vi "PWM Generation.vi"() -> ()   [LabVIEW 2021]
uses:
  <vilib>/myRIO/Instrument Drivers/Onboard IO/DIO/typedefs/DIO Reference.ctl
  <vilib>/myRIO/Common/Instrument Driver Framework/Utilities/typedefs/myRIO Generic Hardware Reference.ctl
  <vilib>/myRIO/Common/Instrument Driver Framework/Utilities/typedefs/Hardware Version Enum.ctl
  <vilib>/myRIO/Common/Instrument Driver Framework/Utilities/typedefs/myRIO v1.0 Reference.ctl
  <vilib>/myRIO/Common/Instrument Driver Framework/Utilities/typedefs/Generic FPGA Reference.ctl
  <vilib>/myRIO/Common/Instrument Driver Framework/myRIO v1.0/DIO/typedefs/DIO Channels List.ctl
  <vilib>/myRIO/Common/Instrument Driver Framework/myRIO v1.0/DIO/typedefs/DIO Channels Enum.ctl
  <vilib>/userDefined/High Color/nirio_resource_hc.ctl
  <vilib>/myRIO/Common/Instrument Driver Framework/Utilities/vis/Is FPGA Ref Available.vi
  <vilib>/myRIO/Common/Instrument Driver Framework/myRIO v1.0/DIO/vis/myRIO v1.1 Open Throughput DIO.vi
  <vilib>/myRIO/Instrument Drivers/Onboard IO/DIO/vis/Write.vi
  <vilib>/myRIO/Common/Instrument Driver Framework/Utilities/vis/Validate Channels.vi
  <vilib>/myRIO/Common/Instrument Driver Framework/myRIO v1.0/DIO/vis/myRIO v1.0 Reserve DIO.vi
  <vilib>/myRIO/Common/Instrument Driver Framework/myRIO v1.0/Resource Manager/vis/myRIO v1.0 Reserve Channel List.vi
  <vilib>/myRIO/Common/Instrument Driver Framework/myRIO v1.0/DIO/vis/myRIO v1.0 Build MUX Configuration DIO.vi
  <vilib>/myRIO/Common/Instrument Driver Framework/myRIO v1.0/Resource Manager/vis/myRIO v1.0 Reserve Channel.vi
  <vilib>/myRIO/Common/Instrument Driver Framework/myRIO v1.0/Resource Manager/vis/myRIO v1.0 Unreserve Channel.vi
  <vilib>/myRIO/Common/Instrument Driver Framework/myRIO v1.0/Resource Manager/vis/myRIO v1.0 Create Configuration List.vi
  <vilib>/myRIO/Common/Instrument Driver Framework/myRIO v1.0/Resource Manager/vis/myRIO v1.0 Build Mutex Name.vi
  <vilib>/Utility/VariantDataType/GetNumericInfo.vi
  <vilib>/Utility/error.llb/Error Cluster From Error Code.vi
  <vilib>/myRIO/Common/Instrument Driver Framework/myRIO v1.0/myRIO v1.1 Open Throughput.vi
  <vilib>/myRIO/Common/Instrument Driver Framework/Utilities/vis/IO Manager.vi
  <vilib>/myRIO/Common/Instrument Driver Framework/Utilities/vis/Configuration Manager.vi
  <vilib>/myRIO/Common/Instrument Driver Framework/myRIO v1.0/Resource Manager/vis/myRIO v1.0 Configure IO.vi
  <vilib>/myRIO/Common/Instrument Driver Framework/myRIO v1.0/myRIO v1.0 Close.vi
  <vilib>/myRIO/Common/Instrument Driver Framework/myRIO v1.0/DIO/vis/myRIO v1.0 Write DIO.vi
  <vilib>/myRIO/Express VI/Onboard Devices/LED/LED Express VI.xnode
  <vilib>/myRIO/Instrument Drivers/Onboard IO/DIO/vis/myRIO DIO Open.xnode
  <vilib>/myRIO/Instrument Drivers/Onboard IO/DIO/DIO.lvlib
panel:
  out "?":bool
  out "?":dbl format="%#_2g"
  out "?":bool
  in  "?":bool
  in  "?":u32=100
  in  "Duty Cycle (%) for PWM 2":dbl(slide)=50.0 caption="Duty Cycle (%)" scale=0.0..100.0
  in  "Frequency for PWM 2":dbl(slide)=10.1 caption="Frequency" scale=0.0..100.0
  in  "Duty Cycle (%) for PWM 1":dbl(slide)=50.0 caption="Duty Cycle (%)" scale=0.0..100.0
  in  "Frequency for PWM 1":dbl(slide)=10.1 caption="Frequency" scale=0.0..100.0
  out "PWM 1":dynamicdata(graph)
  out "PWM 2":dynamicdata(graph)
  # "CONTROL BLINKING LED 0"
  # "CONTROL DIMMING"
  # "PERCENTAGE OF DIMMING :"
  # "Miliseconds to wait"
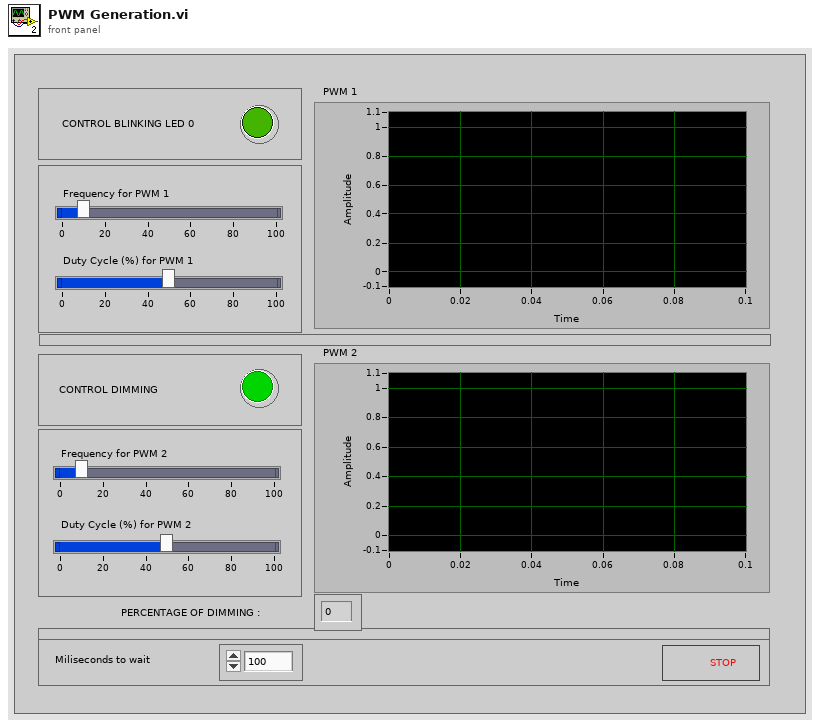
[diagram p1: front panel]
types:
  T1 = typedef "DIO.lvlib/DIO Reference.ctl" = cluster{"myRIO Reference":T2, "DIO Channels List":T6}
  T2 = typedef "myRIO Generic Hardware Reference.ctl" = cluster{"myRIO Model":T3, "myRIO Hardware Reference":T4}
  T3 = typedef "Hardware Version Enum.ctl" = enum16{"Unknown", "myRIO-1900", "myRIO-1950", "roboRIO", "NI ELVIS RIO CM", "ELVIS III"}
  T4 = typedef "myRIO v1.0 Reference.ctl" = cluster{"Generic FPGA Reference":T5, "Allow multiple opens":bool}
  T5 = typedef "Generic FPGA Reference.ctl" = refnum<k20>
  T6 = typedef "DIO Channels List.ctl" = T7[]
  T7 = typedef "DIO Channels Enum.ctl" = enum16{"Not Connected", "C/DIO0", "C/DIO1", "C/DIO2", "C/DIO3", "C/DIO4", "C/DIO5", "C/DIO6", "C/DIO7", "A/DIO0", "A/DIO1", "A/DIO2", "A/DIO3", "A/DIO4", "A/DIO5", "A/DIO6", "A/DIO7", "A/DIO8", "A/DIO9", "A/DIO10", "A/DIO11", "A/DIO12", "A/DIO13", "A/DIO14", "A/DIO15", "A/DIO16", "A/DIO17", "A/DIO18", "A/DIO19", "B/DIO0", "B/DIO1", "B/DIO2", "B/DIO3", "B/DIO4", "B/DIO5", "B/DIO6", "B/DIO7", "B/DIO8", "B/DIO9", "B/DIO10", "B/DIO11", "B/DIO12", "B/DIO13", "B/DIO14", "B/DIO15", "B/DIO16", "B/DIO17", "B/DIO18", "B/DIO19", "LED0", "LED1", "LED2", "LED3", "Button0", "DIO/DIO0", "DIO/DIO1", "DIO/DIO2", "DIO/DIO3", "DIO/DIO4", "DIO/DIO5", "DIO/DIO6", "DIO/DIO7", "DIO/DIO8", "DIO/DIO9", "SPI/CS0", "SPI/CS1", "SPI/CS2", "SPI/CS3", "LED RADIO (Green)", "LED RADIO (Red)", "LED COMM (Green)", "LED COMM (Red)", "LED MODE (Green)", "LED MODE (Red)"}
  T8 = typedef "nirio_resource_hc.ctl" = tag
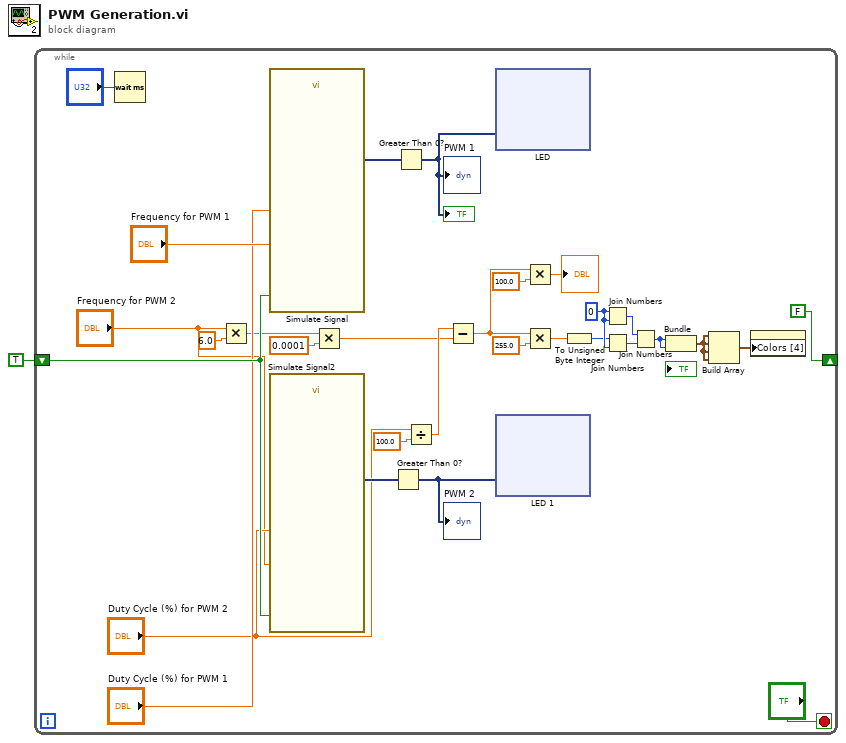
[diagram p0: block diagram]
diagram:
  n1 = while {
    shift-right: [FALSE] -> _
    shift-left: TRUE -> [w25]
    stop <- "?" stop-if-true
    w21 = u8 0 ("lo")
    n2 = Wait (ms)(milliseconds to wait="?") -> ()  [unwired: 1 out]
    n3 = Multiply(x="Frequency for PWM 2", y=6.0) -> (x*y=w12:dbl)
    n4 = call "Simulate Signal"("Duty Cycle (%)"="Duty Cycle (%) for PWM 1", "Reset Signal"=w25, "Frequency"="Frequency for PWM 1") -> ("Square"=w31:dynamicdata)  [unwired: 11 in, 1 out]
    n5 = call "Simulate Signal2"("Duty Cycle (%)"="Duty Cycle (%) for PWM 2", "Reset Signal"=w25, "Frequency"="Frequency for PWM 2") -> ("Square"=w26:dynamicdata)  [unwired: 11 in, 1 out]
    n6 = Multiply(x=w12, y=0.0001) -> (x*y=w9:dbl)
    n7 = Greater Than 0?(x=w26) -> (x > 0?=w24:dynamicdata)
    "PWM 2" <- w24
    n8 = Greater Than 0?(x=w31) -> (x > 0?=w2:dynamicdata)
    "PWM 1" <- w2
    "?" <- w2
    n9 = Divide(x="Duty Cycle (%) for PWM 2", y=100.0) -> (x/y=w10:dbl)
    n10 = Subtract(x=w10, y=w9) -> (x-y=w5:dbl)
    n11 = xnode "LED"("LED0"=w2) -> ()  [unwired: 1 in, 1 out]
    n12 = xnode "LED 1"("LED1"=w24) -> ()  [unwired: 1 in, 1 out]
    n13 = Multiply(x=w5, y=100.0) -> (x*y=→"?":dbl)
    n14 = Multiply(x=w5, y=255.0) -> (x*y=w7:dbl)
    n15 = To Unsigned Byte Integer(number=w7) -> (unsigned 8bit integer=w6:u8)
    n16 = Join Numbers(hi=w21, lo=w21) -> ((hi.lo)=w23:u16)
    n17 = Join Numbers(hi=w6, lo=w21) -> ((hi.lo)=w22:u16)
    n18 = Join Numbers(hi=w23, lo=w22) -> ((hi.lo)=w20:u32)
    n19 = Bundle(w20, w20) -> (w19:cluster{u32, u32})  [unwired: 1 in]
    n20 = Build Array(w19, w19, w19, w19) -> (w18:cluster{u32, u32}[])
    n21 = property class="Bool (strict)"("Colors [4]"=w18) -> ()  [unwired: 2 in, 2 out]
  }
